vi "Check Init Complete.vi"(0 "String":string) -> (4 "Shutdown (T/F)":bool)   [LabVIEW 2020]
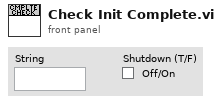
[diagram p1: front panel]
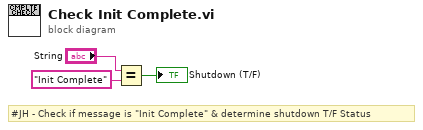
[diagram p0: block diagram]
diagram:
  # "#JH - Check if message is \"Init Complete\" & determine shutdown T/F Status"
  n1 = Equal?(x="String", y="Init Complete") -> (x = y?=→"Shutdown (T/F)":bool)
